vi "Get Run Remote Data.vi"(8 "error in (no error)":errorcluster, 11 "Node Config in":refnum<class "Node Config.lvclass">) -> (0 "error out":errorcluster, 2 "Run Remote Data":bool, 3 "Node Config out":refnum<class "Node Config.lvclass">)   [LabVIEW 2020, in "Vecto.lvlib" / "Node Config.lvclass"]
uses:
  Node Config.lvclass
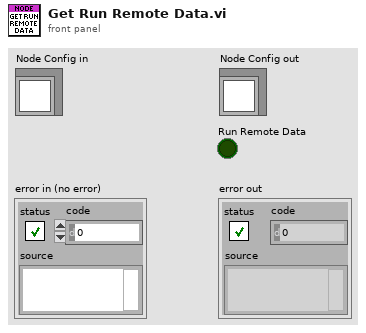
[diagram p1: front panel]
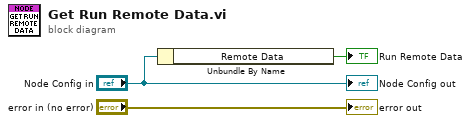
[diagram p0: block diagram]
diagram:
  n1 = Unbundle By Name("Node Config in") -> ("Remote Data"=→"Run Remote Data":bool)
  "error out" <- "error in (no error)"
  "Node Config out" <- "Node Config in"
